vi "Write Charge Pump.vi"(8 "error in (no error)":errorcluster, 10 "Parameter Cluster":T1, 11 "Toggle 6 in":refnum<class "Toggle 6.lvclass">) -> (0 "error out":errorcluster, 3 "Toggle 6 out":refnum<class "Toggle 6.lvclass">)   [LabVIEW 2020, in "Toggle 6.lvclass"]
uses:
  Toggle 6.lvclass
  Controls/Parameter Cluster.ctl
  Toggle 6.lvclass/Toggle 6.ctl
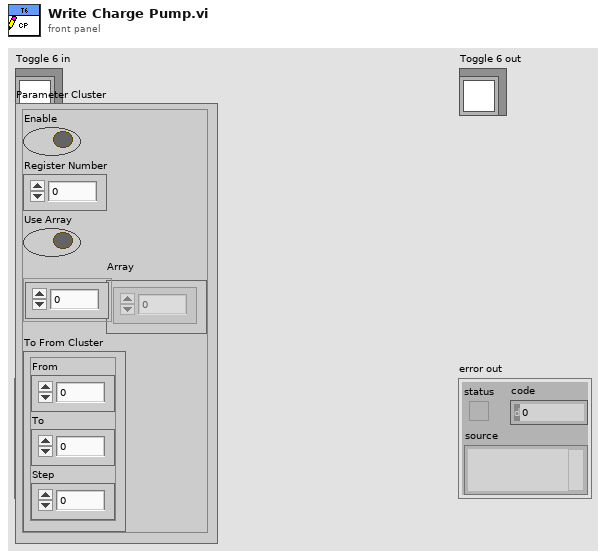
[diagram p1: front panel]
types:
  T1 = typedef "Toggle 6.lvclass/Parameter Cluster.ctl" = cluster{"Enable":bool, "Register Number":u32, "Use Array":bool, "Array":dbl[], "To From Cluster":cluster{"From":dbl, "To":dbl, "Step":dbl}}
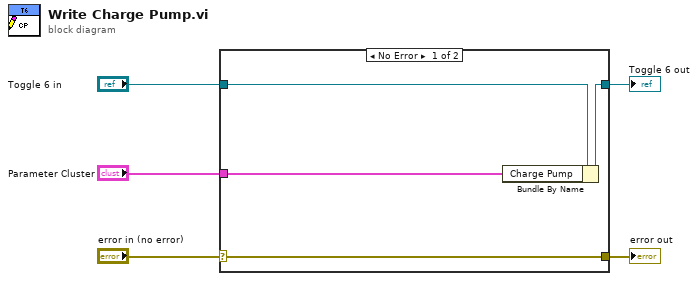
[diagram p0: block diagram]
diagram:
  n1 = case shown="No Error" "error in (no error)" {
    selector: "error in (no error)" -> [w9 w10]
    tunnel: [w9 w10] -> w4
    tunnel: [w7 w11] -> w2
    tunnel: "Toggle 6 in" -> [w8 w11]
    tunnel: "Parameter Cluster" -> [w6 _]
    frame No Error {
      n2 = Bundle By Name(cluster=w8, "Charge Pump"=w6) -> (w7:refnum<class "Toggle 6.lvclass">)
    }
    frame Error {
    }
  }
  "error out" <- w4
  "Toggle 6 out" <- w2
